vi "Actor Core.vi"(8 "error in":errorcluster, 11 "Nested in":refnum<class "QPDController.lvclass">) -> (0 "error out":errorcluster, 3 "Actor out":refnum<class "Actor.lvclass">)   [LabVIEW 2020, in "QPDController.lvlib" / "QPDController.lvclass"]
doc: "(<B>Filename</B>: Actor Framework.lvlib:Actor.lvclass:Actor Core.vi)\n\nReceives messages to the actor, reacts to them, and initiates any error handling that may shut the actor down.\n\nDescendant classes may override this VI to append parallel tasks for the actor to complete while it handles messages. Overrides use the Call Parent Method node."
uses:
  QPDController.lvclass
  <vilib>/ActorFramework/Actor/Actor.lvclass
  <vilib>/ActorFramework/Stop Msg/Stop Msg.lvclass
  Model/Hardware Layer/Real Hardware/DAQ_QPT_Throlab/DAQ_QPT_Throlab Messages/Start TIRF Locked Msg/Start TIRF Locked Msg.lvclass
  Model/Hardware Abstraction Layer/Component/GenericActor/GenericActor/GenericController.lvclass
  E:/Development/DevHardSoftware/MicroscopyFramework/Model/Hardware Abstraction Layer/Component/GenericActor/GenericActor/GenericController.lvclass
  C:/Program Files/National Instruments/LabVIEW 2020/vi.lib/ActorFramework/Actor/Actor.lvclass
  E:/Development/DevHardSoftware/MicroscopyFramework/Interface/DataGenerator/DataGenerator.lvclass
  E:/Development/DevHardSoftware/MicroscopyFramework/Interface/DataListener/DataListener.lvclass
  E:/Development/DevHardSoftware/MicroscopyFramework/Interface/ErrorHandler/ErrorHandler.lvclass
  E:/Development/DevHardSoftware/MicroscopyFramework/ViewController/QPDController/QPDController.lvclass
panel:
  in  "Tirf_Locked":bool
  out "QPD Y":dbl(graph)
  out "QPD X":dbl(graph)
  out "Sum":dbl
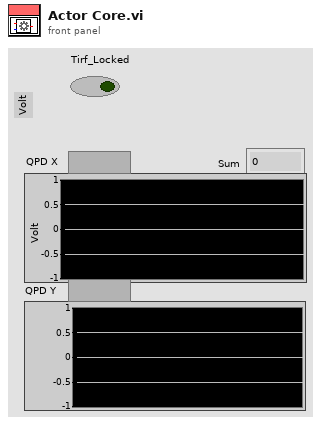
[diagram p1: front panel]
types:
  T1 = cluster{"Stop":refnum<user-event>, "QPD X":refnum<user-event>, "QPD Y":refnum<user-event>, "Sum":refnum<user-event>}
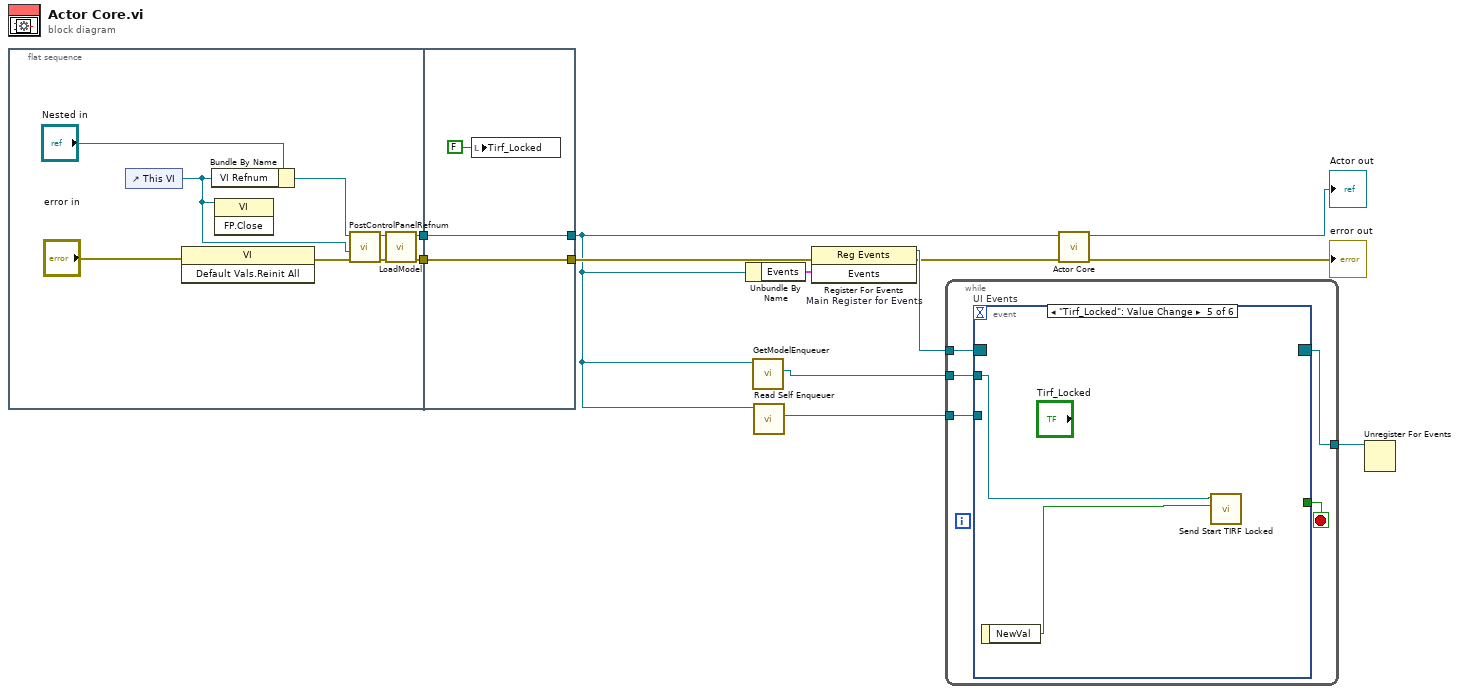
[diagram p0: block diagram]
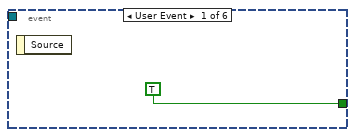
[diagram p2: hidden frame]
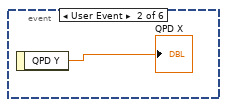
[diagram p3: hidden frame]
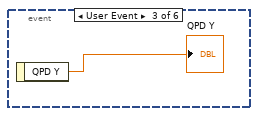
[diagram p4: hidden frame]
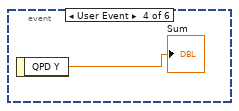
[diagram p5: hidden frame]
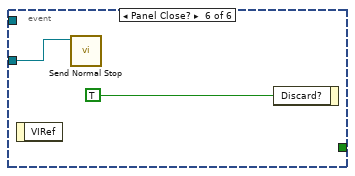
[diagram p6: hidden frame]
diagram:
  n1 = flat-sequence {
    tunnel: [w15] -> w2
    tunnel: [w13] -> w1
    tunnel: [w23] -> w4
    tunnel: [w24] -> w5
    tunnel: w2 -> [w24]
    tunnel: w1 -> [w23]
    frame #0 {
      n2 = control-ref of="This VI"() -> (w16:refnum<vi>)
      n3 = invoke class="VI" method="Default Vals.Reinit All"(error in="error in") -> (error out=w20:errorcluster)  [unwired: 2 in, 2 out]
      n4 = Bundle By Name(cluster="Nested in", "VI Refnum"=w16) -> (w17:refnum<class "QPDController.lvclass">)
      n5 = invoke class="VI" method="FP.Close"(reference=w16) -> ()  [unwired: 2 in, 3 out]
      n6 = call-dynamic "PostControlPanelRefnum.vi"("error in (no error)"=w20, "VI Refnum"=w16, "GRMActor in"=w17) -> ("error out"=w18:errorcluster, "GRMActor out"=w14:refnum<class "QPDController.lvclass">)  [unwired: 7 in]
      n7 = call-dynamic "LoadModel.vi"("error in (no error)"=w18, "GRMActor in"=w14) -> ("error out"=w15:errorcluster, "GRMActor out"=w13:refnum<class "QPDController.lvclass">)  [unwired: 8 in]
    }
    frame #1 {
      n8 = local write "Tirf_Locked"(FALSE ("Tirf_Locked")) -> ()
    }
  }
  n9 = Unbundle By Name(w4) -> ("Events"=w9:T1)
  n10 = call-dynamic "GetModelEnqueuer.vi"("GRMActor in"=w4) -> ("ModelEnqueuer"=w3:refnum<class "Message Enqueuer.lvclass">)  [unwired: 8 in, 2 out]
  n11 = call <vilib>:"Read Self Enqueuer.vi"("Actor"=w4) -> ("Self Enqueuer"=w7:refnum<class "Message Enqueuer.lvclass">)  [unwired: 10 in]
  n12 = register-events "Main Register for Events"(error in=w5, w9) -> (reference out=w10:refnum<event-registration>, error out=w6:errorcluster)  [unwired: 1 in]
  n13 = while {
    tunnel: w10 -> [w29]
    tunnel: [w27] -> w8
    tunnel: w7 -> [w26]
    tunnel: w3 -> [w25]
    stop <- w28 stop-if-true
    n14 = event "UI Events" shown="[4] \"Tirf_Locked\": Value Change" {
      selector: w29 -> [_ _ _ _ _ _]
      dyn-events: [_ _ _ _ _ _] -> w27
      timeout: _ -> [_ _ _ _ _ _]
      tunnel: [TRUE _ _ _ _ _] -> w28
      tunnel: w26 -> [_ _ _ _ _ w36]
      tunnel: w25 -> [_ _ _ _ w35 _]
      event User Event {
        n15 = event-data() -> ()  [unwired: 1 in, 1 out]
      }
      event User Event {
        n16 = event-data() -> ("QPD Y"=→"QPD X":dbl)  [unwired: 1 in]
      }
      event User Event {
        n17 = event-data() -> ("QPD Y"=→"QPD Y":dbl)  [unwired: 1 in]
      }
      event User Event {
        n18 = event-data() -> ("QPD Y"=→"Sum":dbl)  [unwired: 1 in]
      }
      event "Tirf_Locked": Value Change {
        n19 = event-data() -> ("NewVal"=w34:bool)  [unwired: 1 in]
        n20 = call "Send Start TIRF Locked.vi"("TIRF Locked?"=w34, "Message Enqueuer"=w35) -> ()  [unwired: 8 in, 2 out]
      }
      event Panel Close? {
        n21 = event-data() -> ()  [unwired: 1 in, 1 out]
        n22 = call <vilib>:"Send Normal Stop.vi"("Message Enqueuer"=w36) -> ()  [unwired: 10 in, 1 out]
        n23 = event-data("Discard?"=TRUE) -> ()  [unwired: 1 in, 1 out]
      }
    }
  }
  n24 = call-parent "Actor Core.vi"("error in"=w6, "Actor in"=w4) -> ("error out"=→"error out":errorcluster, "Actor out"=→"Actor out":refnum<class "Actor.lvclass">)  [unwired: 8 in]
  n25 = Unregister For Events(event registration refnum=w8) -> ()  [unwired: 1 in, 1 out]
